vi "Flash Title Bar.vi"(7 "flash time (ms) (100)":u32=100, 8 "error in (no error)":errorcluster, 9 "number of flashes (1)":i32=1, 10 "window name (\"\")":string, 11 "window refnum (NaWR)":T1) -> (0 "error out":errorcluster, 3 "window refnum out":T1)   [LabVIEW 2020, in "MacroAssert.lvlib" / "WINUTIL.lvlib"]
doc: "This function will make the title bar of the window named in the 'window name' input, or identified by the 'window refnum' flash once, the state of the title bar changing at the specified rate the given number of times. If 'not a window refnum' is passed in, then the function will use the window name to get a window window refnum. If the window cannot be found, an error will be returned."
uses:
  WINUTIL.lvlib
  Window Refnum.ctl
  user32.dll
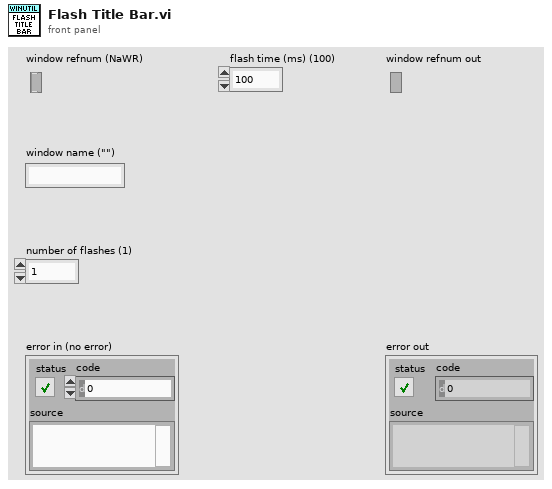
[diagram p1: front panel]
types:
  T1 = typedef "MacroAssert.lvlib/WINUTIL.lvlib/Window Refnum.ctl" = refnum<k1>
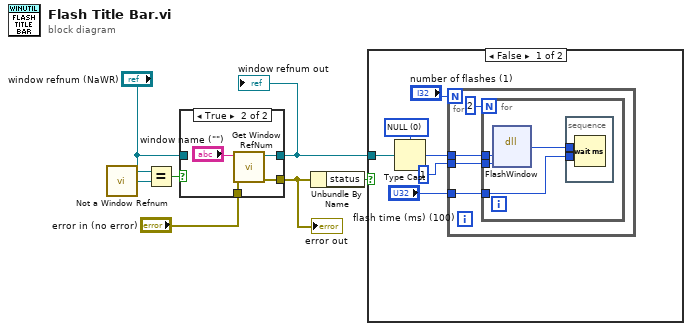
[diagram p0: block diagram]
diagram:
  n1 = call "Not a Window Refnum.vi"() -> ("Not a Window Refnum"=w5:T1)
  n2 = Equal?(x="window refnum (NaWR)", y=w5) -> (x = y?=w6:bool)
  n3 = case shown="True" w6 {
    tunnel: "error in (no error)" -> [w8 w13]
    tunnel: [w9 w12] -> w1
    tunnel: "window refnum (NaWR)" -> [w9 _]
    tunnel: [w8 w11] -> w3
    frame False {
    }
    frame True {
      n4 = call "Get Window RefNum.vi"("error in (no error)"=w13, "window name (\"\")"="window name (\"\")") -> ("error out"=w11:errorcluster, "window refnum (NaWR)"=w12:T1)  [unwired: 8 in]
    }
  }
  "error out" <- w3
  "window refnum out" <- w1
  n5 = Unbundle By Name(w3) -> ("status"=w2:bool)
  n6 = case shown="False" w2 {
    tunnel: w1 -> [w19 _]
    frame False {
      w18 = u32 0 items=["NULL"]
      n7 = Type Cast(type=w18, x=w19) -> (*(type *) &x=w17:u32)
      n8 = for {
        N: "number of flashes (1)" -> [_]
        tunnel: "flash time (ms) (100)" -> [w22]
        tunnel: 1 -> [w21]
        tunnel: w17 -> [w20]
        n9 = for {
          N: 2 -> [_]
          tunnel: w22 -> [w27]
          tunnel: w21 -> [w26]
          tunnel: w20 -> [w25]
          n10 = dll-call lib="USER32.DLL" fn="FlashWindow"("hWnd"=w25, "fInvert"=w26) -> ("active?"=w24:i32)  [unwired: 5 in, 2 out]
          n11 = stacked-sequence {
            tunnel: w27 -> [w28]
            tunnel: w24 -> [_]
            frame #0 {
              n12 = Wait (ms)(milliseconds to wait=w28) -> ()  [unwired: 1 out]
            }
          }
        }
      }
    }
    frame True {
    }
  }
